vi "CONST DI TaskIO KeyName.vi"(6 "DI TaskName":string) -> (7 "DI TaskIO (KeyName)":string)   [LabVIEW 2017, in "DAQ.lvclass"]
doc: "Developed by Kevin Thompson\nkevin@thompsonengineering.net\n\nCopyright 2018-2020\nThompson Engineering, LLC"
uses:
  DAQ.lvclass
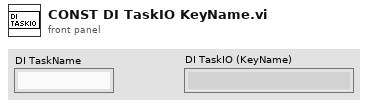
[diagram p1: front panel]
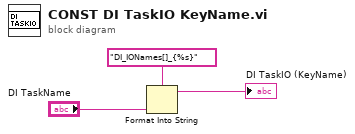
[diagram p0: block diagram]
diagram:
  n1 = Format Into String(format string="DI_IONames[]_{%s}" ("string"), "DI TaskName") -> (resulting string=→"DI TaskIO (KeyName)":string)  [unwired: 2 in, 1 out]
